vi "MultithreadedUDPReadWriteAnalyze.vi"() -> ()   [LabVIEW 2012]
panel:
  out "regmap":string
  out "power monitoring \ndata string":string
  out "UDP Send Error Initialize":errorcluster
  out "Fresh Register map":bool
  out "Last Command Sent":string
  out "UDP Send Error":errorcluster
  out "Original Register Map":string
  out "Register Map":string
  in  "stop":bool
  out "NumBins":u32
  out "Cnts/Bin":u32
  out "Prof/Hist":u32
  out "Sync":u32
  out "Channel":u32
  out "rTime":u32
  out "frameCntr":u32
  out "UDP Close Error":errorcluster
  out "Profile Byte by Byte":u8[](graph)
  out "Profile":u32[](graph)
  in  "Profile Number":u32
  out "Queue close error":errorcluster
  out "Queue Add Data Error":errorcluster
  out "Queue creation error":errorcluster
  out "UDP Read Error":errorcluster
  in  "port":u16=24599
  out "UDP Open Error":errorcluster
  # "0\n1\n2\n3\n4\n5\n6\n7\n8\n9\n10\n11"
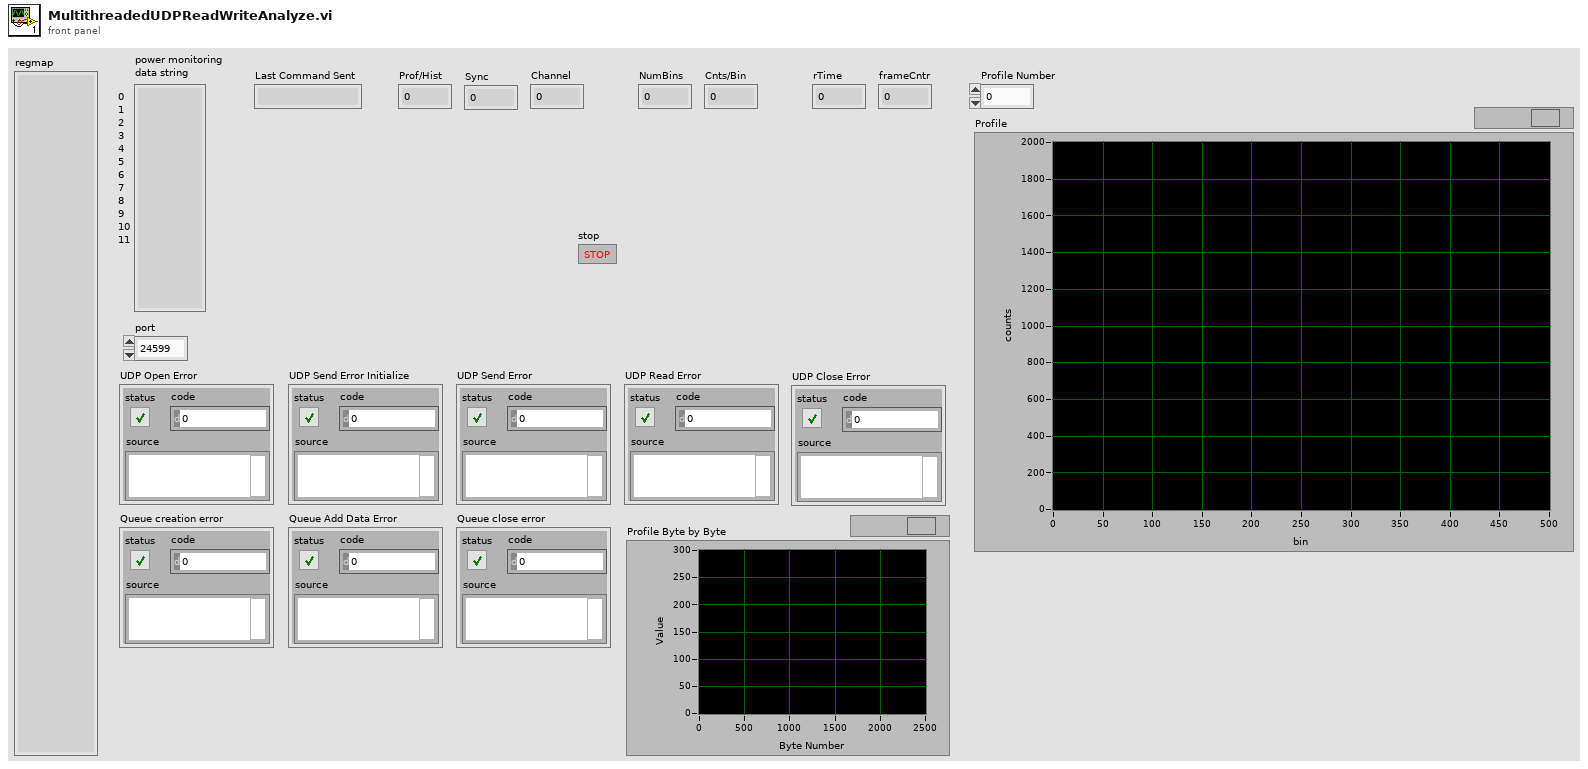
[diagram p1: front panel]
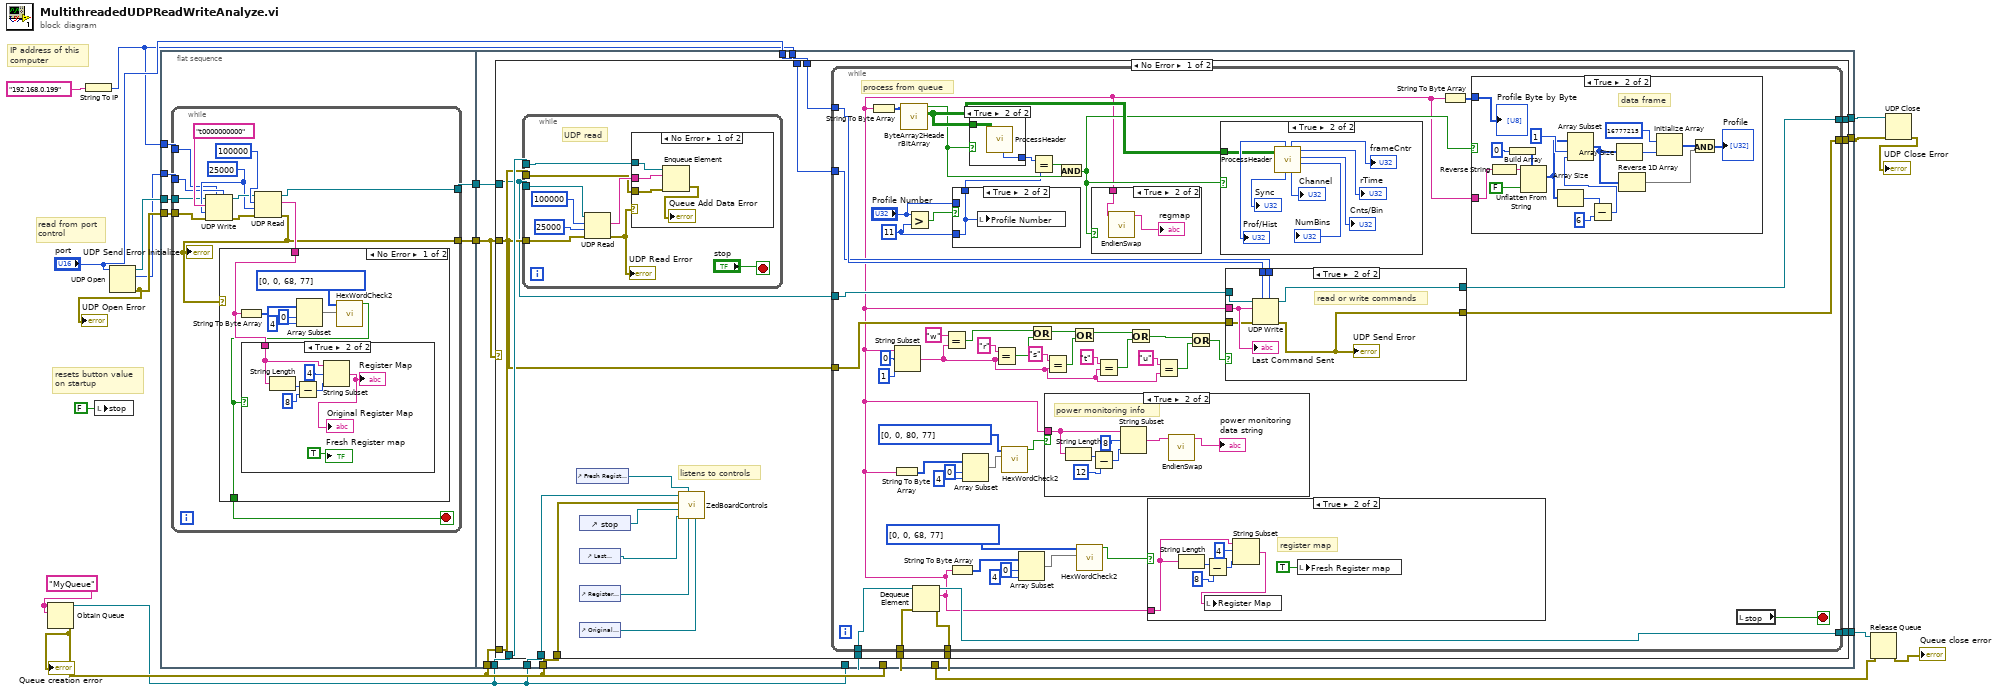
[diagram p0: block diagram]
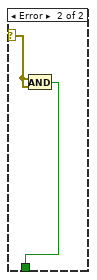
[diagram p3: hidden frame]
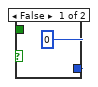
[diagram p9: hidden frame]
diagram:
  w17 = "MyQueue" ("name (unnamed)")
  # "IP address of this \ncomputer"
  # "resets button value \non startup"
  # "read from port\ncontrol"
  n1 = Obtain Queue(name (unnamed)=w17, element data type=w17) -> (queue out=w8:refnum<queue>, error out=w9:errorcluster)  [unwired: 3 in, 1 out]
  "Queue creation error" <- w9
  n2 = String To IP(1:"192.168.0.199" ("name")) -> (0:w3:u32)
  n3 = local write "stop"(FALSE ("stop")) -> ()
  n4 = UDP Open(11:"port") -> (port=w6:refnum<k16>, 0:w7:errorcluster, 2:w4:u16)  [unwired: 4 in]
  "UDP Open Error" <- w7
  n5 = flat-sequence {
    tunnel: w7 -> [w24]
    tunnel: w6 -> [w23]
    tunnel: w4 -> [w22]
    tunnel: w3 -> [w21]
    tunnel: [w20] -> w2
    tunnel: [w19] -> w1
    tunnel: w8 -> [w67]
    tunnel: w9 -> [w66]
    tunnel: w8 -> [w65]
    tunnel: [w64] -> w13
    tunnel: [w63] -> w12
    tunnel: w9 -> [w62]
    tunnel: [w61] -> w11
    tunnel: [w60] -> w10
    tunnel: w3 -> [w59]
    tunnel: "port" -> [w58]
    tunnel: w9 -> [w57]
    tunnel: w8 -> [w56]
    tunnel: w2 -> [w55]
    tunnel: w1 -> [w54]
    frame #0 {
      n6 = while {
        tunnel: w24 -> [w29]
        tunnel: w23 -> [w30]
        tunnel: w22 -> [w32]
        tunnel: w21 -> [w31]
        tunnel: [w27] -> w20
        tunnel: [w26] -> w19
        stop <- w25 stop-if-true
        w33 = 25000 ("timeout ms (25000)")
        n7 = UDP Write(address=w31, port or service name=w32, connection ID=w30, data in="t0000000000", 8:w29, 9:w33) -> (error out=w36:errorcluster, 3:w35:refnum<k16>)
        n8 = UDP Read(connection ID=w35, max size (548)=100000, timeout ms (25000)=w33, 8:w36) -> (data out=w28:string, error out=w26:errorcluster, 3:w27:refnum<k16>)  [unwired: 2 out]
        "UDP Send Error Initialize" <- w26
        n9 = case shown="No Error" w26 {
          selector: w26 -> [_ w53]
          tunnel: w28 -> [w39 _]
          tunnel: [w38 w52] -> w25
          frame No Error {
            n10 = String To Byte Array(string=w39) -> (unsigned byte array=w41:u8[])
            n11 = Array Subset(array=w41, index=0, length=4) -> (w42:u8[])
            n12 = call "HexWordCheck2.vi"("array"=w42, "Input Array"=u8[] [0, 0, 68, 77]) -> ("Boolean"=w38:bool)  [unwired: 9 in]
            n13 = case shown="True" w38 {
              tunnel: w39 -> [_ w45]
              frame False {
              }
              frame True {
                n14 = String Length(string=w45) -> (length=w49:i32)
                n15 = Subtract(x=w49, y=8) -> (x-y=w51:i32)
                n16 = String Subset(string=w45, offset (0)=4, length (rest)=w51) -> (substring=→"Register Map" →"Original Register Map":string)
                "Fresh Register map" <- TRUE ("Fresh Register map")
              }
            }
          }
          frame Error {
            n17 = And(x=w53, y=w53) -> (x .and. y?=w52:bool)
          }
        }
      }
    }
    frame #1 {
      n18 = case shown="No Error" w54 {
        tunnel: w67 -> [w81 _]
        tunnel: w66 -> [w80 w207]
        tunnel: w65 -> [w79 _]
        tunnel: [w78 w208] -> w64
        tunnel: [w77 w209] -> w63
        tunnel: w62 -> [w76 _]
        tunnel: [w75 w207] -> w61
        tunnel: [w74 w210] -> w60
        tunnel: w59 -> [w73 _]
        tunnel: w58 -> [w72 _]
        tunnel: w57 -> [w71 _]
        tunnel: w54 -> [w70 w209]
        tunnel: w56 -> [w69 w210]
        tunnel: w55 -> [w68 w208]
        frame No Error {
          # "listens to controls"
          n19 = while {
            tunnel: w81 -> [w197]
            tunnel: w80 -> [w198]
            tunnel: w70 -> [w200]
            tunnel: w68 -> [w194]
            stop <- "stop" stop-if-true
            # "UDP read"
            n20 = UDP Read(connection ID=w194, max size (548)=100000, timeout ms (25000)=25000, 8:w200) -> (data out=w199:string, error out=w196:errorcluster)  [unwired: 3 out]
            "UDP Read Error" <- w196
            n21 = case shown="No Error" w196 {
              tunnel: w199 -> [w206 _]
              tunnel: w198 -> [w205 _]
              tunnel: w197 -> [w204 _]
              frame No Error {
                n22 = Enqueue Element(queue=w204, element=w206, error in (no error)=w205) -> (error out=→"Queue Add Data Error":errorcluster)  [unwired: 1 in, 2 out]
              }
              frame Error {
              }
            }
          }
          n23 = control-ref of="Fresh Register map"() -> (w86:refnum<vi>)
          n24 = control-ref of="stop"() -> (w84:refnum<vi>)
          n25 = control-ref of="Last Command Sent"() -> (w85:refnum<vi>)
          n26 = control-ref of="Register Map"() -> (w82:refnum<vi>)
          n27 = control-ref of="Original Register Map"() -> (w83:refnum<vi>)
          n28 = call "ZedBoardControls.vi"("Register Map\nDefaults"=w83, "Register Map\nRead Ref"=w82, "NewRegMapReady"=w86, "Last Command\nSent Ref"=w85, "Stop Loop \nRef"=w84, "error out"=w71, "queue out"=w79) -> ()  [unwired: 5 in]
          n29 = while {
            tunnel: w76 -> [w138]
            tunnel: [w136] -> w74
            tunnel: [w137] -> w75
            tunnel: [w132] -> w78
            tunnel: [w131] -> w77
            tunnel: w70 -> [w133]
            tunnel: w73 -> [w135]
            tunnel: w72 -> [w134]
            tunnel: w69 -> [w129]
            tunnel: w68 -> [w128]
            stop <- w130 stop-if-true
            w89 = u32 11 ("y")
            # "process from queue"
            n30 = Greater?(x="Profile Number", y=w89) -> (0:w90:bool)
            n31 = Dequeue Element(queue=w129, error in (no error)=w138) -> (queue out=w136:refnum<queue>, element=w106:string, error out=w137:errorcluster)  [unwired: 1 in, 1 out]
            n32 = String To Byte Array(string=w106) -> (unsigned byte array=w120:u8[])
            n33 = String To Byte Array(string=w106) -> (unsigned byte array=w113:u8[])
            n34 = String Subset(string=w106, offset (0)=0, length (rest)=1 ("length (rest)")) -> (substring=w101:string)
            n35 = call "ByteArray2HeaderBitArray.vi"("Input Byte Array"=w120) -> ("Header Array"=w110:bool[][], "Found Header"=w91:bool)  [unwired: 9 in]
            n36 = Equal?(x="w", y=w101) -> (x = y?=w100:bool)
            n37 = String To Byte Array(string=w106) -> (unsigned byte array=w107:u8[])
            n38 = case shown="True" w90 {
              tunnel: w89 -> [_ w140]
              tunnel: [w139 w140] -> w88
              tunnel: "Profile Number" -> [w139 _]
              frame False {
              }
              frame True {
                n39 = local write "Profile Number"(w140) -> ()
              }
            }
            n40 = Array Subset(array=w113, index=0, length=4) -> (w112:u8[])
            n41 = case shown="True" w91 {
              tunnel: w110 -> [_ w177]
              tunnel: [u32 0 ("Channel") w176] -> w122
              frame False {
              }
              frame True {
                n42 = call "ProcessHeader.vi"("Array"=w177) -> ("Channel"=w176:u32)  [unwired: 4 in, 6 out]
              }
            }
            n43 = Equal?(x="r" ("y"), y=w101) -> (x = y?=w99:bool)
            n44 = call "HexWordCheck2.vi"("array"=w112, "Input Array"=u8[] [0, 0, 80, 77] ("array")) -> ("Boolean"=w111:bool)  [unwired: 9 in]
            n45 = Array Subset(array=w107, index=0, length=4) -> (w108:u8[])
            n46 = Or(x=w100, y=w99) -> (x .or. y?=w98:bool)
            n47 = Equal?(x=w122, y=w88) -> (x = y?=w121:bool)
            n48 = Equal?(x="s" ("y"), y=w101) -> (x = y?=w97:bool)
            n49 = case shown="True" w111 {
              tunnel: w106 -> [_ w145]
              frame False {
              }
              frame True {
                # "power monitoring info"
                n50 = String Length(string=w145) -> (length=w146:i32)
                n51 = Subtract(x=w146, y=12) -> (x-y=w148:i32)
                n52 = String Subset(string=w145, offset (0)=8, length (rest)=w148) -> (substring=w144:string)
                n53 = call "EndienSwap.vi"("name (unnamed)"=w144) -> ("concatenated string"=→"power monitoring \ndata string":string)  [unwired: 10 in]
              }
            }
            n54 = And(x=w121, y=w91) -> (x .and. y?=w109:bool)
            n55 = Or(x=w98, y=w97) -> (x .or. y?=w96:bool)
            n56 = call "HexWordCheck2.vi"("array"=w108, "Input Array"=u8[] [0, 0, 68, 77] ("array")) -> ("Boolean"=w126:bool)  [unwired: 9 in]
            n57 = case shown="True" w109 {
              tunnel: w106 -> [_ w141]
              frame False {
              }
              frame True {
                n58 = call "EndienSwap.vi"("name (unnamed)"=w141) -> ("concatenated string"=→"regmap":string)  [unwired: 10 in]
              }
            }
            n59 = Equal?(x="t" ("y"), y=w101) -> (x = y?=w95:bool)
            n60 = Or(x=w96, y=w95) -> (x .or. y?=w94:bool)
            n61 = case shown="True" w126 {
              tunnel: w106 -> [_ w190]
              frame False {
              }
              frame True {
                # "register map"
                n62 = String Length(string=w190) -> (length=w193:i32)
                n63 = Subtract(x=w193, y=8) -> (x-y=w192:i32)
                n64 = String Subset(string=w190, offset (0)=4, length (rest)=w192) -> (substring=w191:string)
                n65 = local write "Register Map"(w191) -> ()
                n66 = local write "Fresh Register map"(TRUE ("Fresh Register map")) -> ()
              }
            }
            n67 = Equal?(x="u" ("y"), y=w101) -> (x = y?=w93:bool)
            n68 = Or(x=w94, y=w93) -> (x .or. y?=w92:bool)
            n69 = case shown="True" w109 {
              tunnel: w110 -> [_ w168]
              frame False {
              }
              frame True {
                n70 = call "ProcessHeader.vi"("Array"=w168) -> ("Number of Bins"=→"NumBins":u32, "Counts Per Bin"=→"Cnts/Bin":u32, "rTime"=→"rTime":u32, "Channel"=→"Channel":u32, "Frame Counter"=→"frameCntr":u32, "Sync"=→"Sync":u32, "Profiles Per Hist"=→"Prof/Hist":u32)  [unwired: 4 in]
              }
            }
            n71 = case shown="True" w92 {
              tunnel: w106 -> [_ w186]
              tunnel: w135 -> [_ w185]
              tunnel: w134 -> [_ w184]
              tunnel: w128 -> [w179 w183]
              tunnel: w133 -> [w178 w182]
              tunnel: [w179 w181] -> w132
              tunnel: [w178 w180] -> w131
              frame False {
              }
              frame True {
                # "read or write commands"
                n72 = UDP Write(address=w185, port or service name=w184, connection ID=w183, data in=w186, 8:w182) -> (error out=w180:errorcluster, 3:w181:refnum<k16>)  [unwired: 1 in]
                "UDP Send Error" <- w180
                "Last Command Sent" <- w186
              }
            }
            n73 = String To Byte Array(string=w106) -> (unsigned byte array=w119:u8[])
            n74 = case shown="True" w109 {
              tunnel: w119 -> [_ w152]
              tunnel: w106 -> [_ w151]
              frame False {
              }
              frame True {
                # "data frame"
                n75 = Reverse String(1:w151) -> (0:w160:string)
                n76 = Build Array(u32 0) -> (w154:u32[])
                n77 = Unflatten From String(type=w154, binary string=w160, data includes array or string size? (T)=FALSE) -> (value=w156:u32[])  [unwired: 2 in, 2 out]
                n78 = Array Size(array=w156) -> (size(s)=w157:i32)
                n79 = Subtract(x=w157, y=6) -> (x-y=w150:i32)
                n80 = Array Subset(array=w156, index=1, length=w150) -> (w161:u32[])
                n81 = Array Size(array=w161) -> (size(s)=w164:i32)
                n82 = Reverse 1D Array(array=w161) -> (reversed array=w162:u32[])
                n83 = Initialize Array(u32 16777215 ("x*2^n"), w164) -> (w163:u32[])
                n84 = And(x=w163, y=w162) -> (x .and. y?=→"Profile":u32[])
                "Profile Byte by Byte" <- w152
              }
            }
            n85 = local read "stop"() -> (w130:bool)
          }
        }
        frame Error {
        }
      }
    }
  }
  n86 = Release Queue(queue=w10, error in (no error)=w11) -> (error out=→"Queue close error":errorcluster)  [unwired: 1 in, 2 out]
  n87 = UDP Close(connection ID=w13, 8:w12) -> (error out=→"UDP Close Error":errorcluster)  [unwired: 1 out]
